vi "FestoCPX.Station.ProdPresent.CheckID.vi"(6 "Max Stab time [ms] (1000)":u32=1000, 7 "SuckerID (0: Final)":i32, 8 "error in":errorcluster) -> (0 "error out":errorcluster, 1 "Present.OK":cluster{"A":bool, "B":bool}, 2 "Present.Final":cluster{"A":bool, "B":bool}, 3 "Present.SuckerID":cluster{"A":bool, "B":bool})   [LabVIEW 2016]
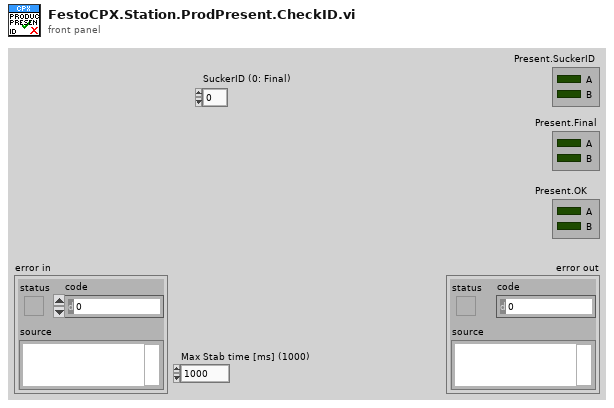
[diagram p1: front panel]
types:
  T1 = typedef "FestoCPX.Station.ProdPresent.ctl" = cluster{"Slot1":cluster{"A":bool, "B":bool}, "Slot2":cluster{"A":bool, "B":bool}, "Slot3":cluster{"A":bool, "B":bool}, "Slot4":cluster{"A":bool, "B":bool}, "Final":cluster{"A":bool, "B":bool}, "OK":cluster{"A":bool, "B":bool}, "Container":cluster{"OK":bool, "NOK":bool}}
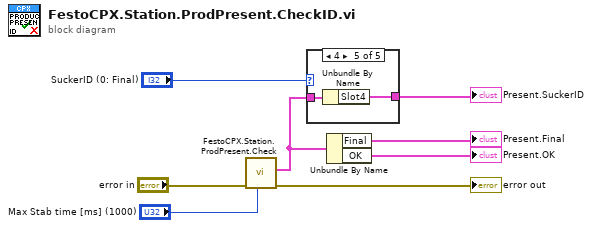
[diagram p0: block diagram]
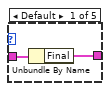
[diagram p2: hidden frame]
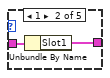
[diagram p3: hidden frame]
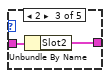
[diagram p4: hidden frame]
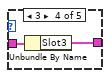
[diagram p5: hidden frame]
diagram:
  n1 = call "FestoCPX.Station.ProdPresent.Check.vi"("Max Stab time [ms] (1000)"="Max Stab time [ms] (1000)", "error in"="error in") -> ("error out"=→"error out":errorcluster, "Prod Present"=w4:T1)  [unwired: 4 in, 4 out]
  n2 = case shown="4" "SuckerID (0: Final)" {
    tunnel: w4 -> [w10 w12 w14 w16 w18]
    tunnel: [w9 w11 w13 w15 w17] -> w5
    frame Default {
      n3 = Unbundle By Name(w10) -> ("Final"=w9:cluster{"A":bool, "B":bool})
    }
    frame 1 {
      n4 = Unbundle By Name(w12) -> ("Slot1"=w11:cluster{"A":bool, "B":bool})
    }
    frame 2 {
      n5 = Unbundle By Name(w14) -> ("Slot2"=w13:cluster{"A":bool, "B":bool})
    }
    frame 3 {
      n6 = Unbundle By Name(w16) -> ("Slot3"=w15:cluster{"A":bool, "B":bool})
    }
    frame 4 {
      n7 = Unbundle By Name(w18) -> ("Slot4"=w17:cluster{"A":bool, "B":bool})
    }
  }
  "Present.SuckerID" <- w5
  n8 = Unbundle By Name(w4) -> ("Final"=→"Present.Final":cluster{"A":bool, "B":bool}, "OK"=→"Present.OK":cluster{"A":bool, "B":bool})
